vi "Create IHandleUnsubscribed.vi"(8 "error in (no error)":errorcluster, 11 "IWampMessage":refnum<class "IWampMessage.lvclass">) -> (0 "error out":errorcluster, 3 "IHandledUnsubscribed out":refnum<class "IHandledUnsubscribed.lvclass">)   [LabVIEW 2020, in "wamplv.lvlib"]
uses:
  wamplv.lvlib
  SerialisedMessages/JSONMessage/JSONMessage.lvclass
  IJsonMessageHandler/IJsonMessageHandler.lvclass
  SerialisedMessages/MsgPackMessage/MsgPackMessage.lvclass
  IMsgPackMessageHandler/IMsgPackMessageHandler.lvclass
  SerialisedMessages/IWampMessage/IWampMessage.lvclass
  IHandleUnsubscribed JSON/IHandleUnsubscribed JSON.lvclass
  C:/local/wamplv/Private/Requests/MessageReceivedHandlers/IJsonMessageHandler/IJsonMessageHandler.lvclass
  C:/local/wamplv/Private/Requests/MessageReceivedHandlers/IReceivedMessageHandler/IReceivedMessageHandler.lvclass
  C:/local/wamplv/Private/Requests/IInternalRequest.lvclass
  C:/local/wamplv/Private/Requests/MessageReceivedHandlers/Unsubscribed/IHandledUnsubscribed/IHandledUnsubscribed.lvclass
  C:/local/wamplv/Private/Requests/MessageReceivedHandlers/Unsubscribed/IHandleUnsubscribed JSON/IHandleUnsubscribed JSON.lvclass
  IHandleUnsubscribed MsgPack/IHandleUnsubscribed MsgPack.lvclass
  C:/local/wamplv/Private/Requests/MessageReceivedHandlers/IMsgPackMessageHandler/IMsgPackMessageHandler.lvclass
  C:/local/wamplv/Private/Requests/MessageReceivedHandlers/Unsubscribed/IHandleUnsubscribed MsgPack/IHandleUnsubscribed MsgPack.lvclass
  IHandledUnsubscribed/IHandledUnsubscribed.lvclass
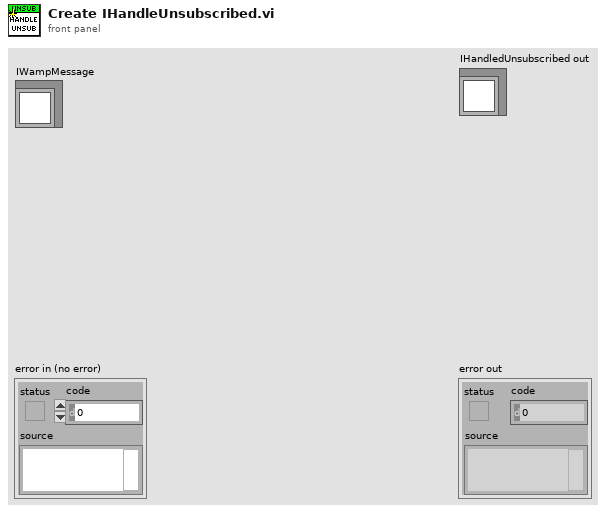
[diagram p1: front panel]
types:
  T1 = typedef "wamplv.lvlib/WAMP Client.lvclass/Serialisation.ctl" = enum16{"JSON", "MessagePack"}
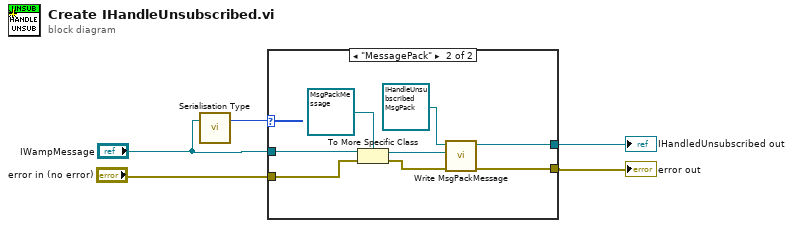
[diagram p0: block diagram]
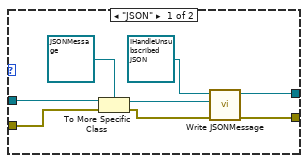
[diagram p2: hidden frame]
diagram:
  n1 = call-dynamic "Serialisation Type.vi"("IWampMessage in"="IWampMessage") -> ("Serialisation Type"=w5:T1)  [unwired: 2 in]
  n2 = case shown="\"MessagePack\"" w5 {
    tunnel: "IWampMessage" -> [w13 w21]
    tunnel: "error in (no error)" -> [w11 w20]
    tunnel: [w7 w15] -> w1
    tunnel: [w8 w16] -> w2
    frame "JSON" {
      n3 = To More Specific Class(target class=refnum<class "JSONMessage.lvclass"> refnum ("wamplv.lvlib:JSONMessage.lvclass"), reference=w13, error in=w11) -> (specific class reference=w10:refnum<class "JSONMessage.lvclass">, error out=w9:errorcluster)
      n4 = call "Write JSONMessage.vi"("error in (no error)"=w9, "wamplv.lvlib:JSONMessage.lvclass"=w10, "IJsonMessageHandler in"=refnum<class "IHandleUnsubscribed JSON.lvclass"> refnum ("wamplv.lvlib:IHandleUnsubscribed JSON.lvclass")) -> ("error out"=w8:errorcluster, "IJsonMessageHandler out"=w7:refnum<class "IHandleUnsubscribed JSON.lvclass">)  [unwired: 7 in]
    }
    frame "MessagePack" {
      n5 = To More Specific Class(target class=refnum<class "MsgPackMessage.lvclass"> refnum ("wamplv.lvlib:MsgPackMessage.lvclass"), reference=w21, error in=w20) -> (specific class reference=w18:refnum<class "MsgPackMessage.lvclass">, error out=w17:errorcluster)
      n6 = call "Write MsgPackMessage.vi"("error in (no error)"=w17, "wamplv.lvlib:MsgPackMessage.lvclass"=w18, "IMsgPackMessageHandler in"=refnum<class "IHandleUnsubscribed MsgPack.lvclass"> refnum ("wamplv.lvlib:IHandleUnsubscribed MsgPack.lvclass")) -> ("error out"=w16:errorcluster, "IMsgPackMessageHandler out"=w15:refnum<class "IHandleUnsubscribed MsgPack.lvclass">)  [unwired: 7 in]
    }
  }
  "error out" <- w2
  "IHandledUnsubscribed out" <- w1
